vi "test_client.vi"() -> ()   [LabVIEW 2017, in "tcp_server.lvlib"]
uses:
  tcp_server.lvlib
panel:
  out "data out":string
  in  "data in":string
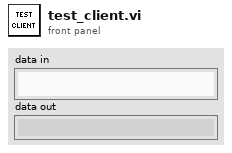
[diagram p1: front panel]
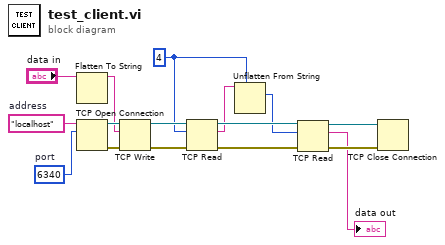
[diagram p0: block diagram]
diagram:
  w5 = 4 ("bytes to read")
  w15 = u16 6340  # port
  w16 = "localhost"  # address
  n1 = Flatten To String(anything="data in") -> (data string=w11:string)  [unwired: 3 in, 2 out]
  n2 = TCP Open Connection(address=w16, remote port or service name=w15) -> (connection ID=w13:refnum<k5>, error out=w14:errorcluster)  [unwired: 3 in]
  n3 = TCP Write(connection ID=w13, data in=w11, error in (no error)=w14) -> (connection ID out=w9:refnum<k5>, error out=w10:errorcluster)  [unwired: 1 in, 1 out]
  n4 = TCP Read(connection ID=w9, bytes to read=w5, error in (no error)=w10) -> (connection ID out=w7:refnum<k5>, data out=w6:string, error out=w8:errorcluster)  [unwired: 2 in]
  n5 = Unflatten From String(type=w5, binary string=w6) -> (value=w4:i32)  [unwired: 3 in, 2 out]
  n6 = TCP Read(connection ID=w7, bytes to read=w4, error in (no error)=w8) -> (connection ID out=w2:refnum<k5>, data out=→"data out":string, error out=w3:errorcluster)  [unwired: 2 in]
  n7 = TCP Close Connection(connection ID=w2, error in (no error)=w3) -> ()  [unwired: 1 in, 2 out]
